vi "Auto_timed_strafe.vi"(3 "Strafe Speed":dbl, 4 "Strafe Time":dbl, 5 "RobotDriveDevRef in":T1) -> (2 "RobotDriveDevRef out":T1)   [LabVIEW 2017]
uses:
  <vilib>/Rock Robotics/WPI/RobotDrive/WPI_RobotDriveDevRef.ctl
  <vilib>/Rock Robotics/WPI/MotorControl/WPI_MotorControlDeviceRef.ctl
  <vilib>/Rock Robotics/WPI/MotorControl/WPI_MotorControlType.ctl
  <vilib>/Rock Robotics/SystemInterfaces/DIO/FPGA_DIOPWMChannel.ctl
  <vilib>/Rock Robotics/WPI/PWM/WPI_PWMDeadband.ctl
  <vilib>/Rock Robotics/SystemInterfaces/DIO/FPGA_DIOChannel.ctl
  <vilib>/Rock Robotics/WPI/RobotDrive/WPI_RobotDriveArcadeDrive_Standard(NoSaturation).vi
  <vilib>/Rock Robotics/Network Tables/NT Write Number.vi
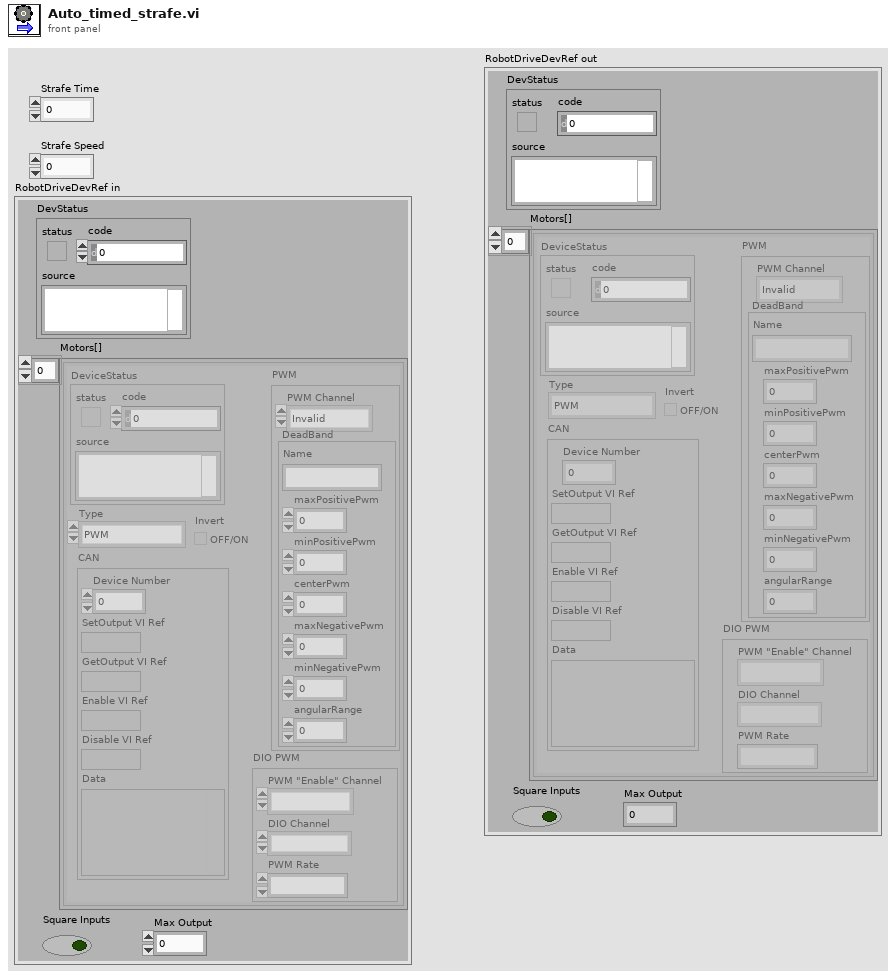
[diagram p1: front panel]
types:
  T1 = typedef "WPI_RobotDriveDevRef.ctl" = cluster{"DevStatus":errorcluster, "Motors[]":T2[], "Square Inputs":bool, "Max Output":dbl}
  T2 = typedef "WPI_MotorControlDeviceRef.ctl" = cluster{"DeviceStatus":errorcluster, "Type":T3, "PWM":cluster{"PWM Channel":T4, "DeadBand":T5}, "CAN":cluster{"Device Number":u8, "SetOutput VI Ref":variant, "GetOutput VI Ref":variant, "Enable VI Ref":variant, "Disable VI Ref":variant, "Data":variant}, "Invert":bool, "DIO PWM":cluster{"PWM \"Enable\" Channel":T4, "DIOChannel":T6, "PWM Rate":dbl}}
  T3 = typedef "WPI_MotorControlType.ctl" = enum16{"PWM", "CAN", "DIO PWM"}
  T4 = typedef "FPGA_DIOPWMChannel.ctl" = enum8{"PWM 0", "PWM 1", "PWM 2", "PWM 3", "PWM 4", "PWM 5", "PWM 6", "PWM 7", "PWM 8", "PWM 9", "PWM MXP 0", "PWM MXP 1", "PWM MXP 2", "PWM MXP 3", "PWM MXP 4", "PWM MXP 5", "PWM MXP 6", "PWM MXP 7", "PWM MXP 8", "PWM MXP 9", "Invalid"}
  T5 = typedef "WPI_PWMDeadband.ctl" = cluster{"Name":string, "maxPositivePwm":i32, "minPositivePwm":i32, "centerPwm":i32, "maxNegativePwm":i32, "minNegativePwm":i32, "angularRange":u16}
  T6 = typedef "FPGA_DIOChannel.ctl" = enum8{"DIO 0", "DIO 1", "DIO 2", "DIO 3", "DIO 4", "DIO 5", "DIO 6", "DIO 7", "DIO 8", "DIO 9", "DIO MXP 0", "DIO MXP 1", "DIO MXP 2", "DIO MXP 3", "DIO MXP 4", "DIO MXP 5", "DIO MXP 6", "DIO MXP 7", "DIO MXP 8", "DIO MXP 9", "DIO MXP 10", "DIO MXP 11", "DIO MXP 12", "DIO MXP 13", "DIO MXP 14", "DIO MXP 15", "SPI Port CS1", "SPI Port CS2", "SPI Port CS3", "SPI Port MISO", "SPI Port MOSI", "Invalid"}
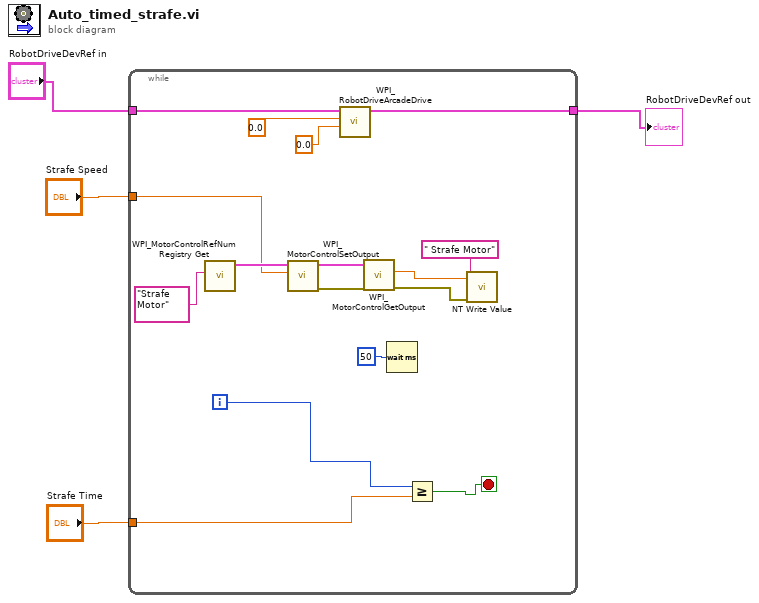
[diagram p0: block diagram]
diagram:
  n1 = while {
    tunnel: "Strafe Speed" -> [w11]
    tunnel: "Strafe Time" -> [w9]
    tunnel: "RobotDriveDevRef in" -> [w6]
    tunnel: [w5] -> w1
    i -> [w10]
    stop <- w20 stop-if-true
    n2 = call <vilib>:"WPI_MotorControlRefNum Registry Get.vi"("refnum name"="Strafe Motor") -> ("MotorControlDevRef"=w17:T2)  [unwired: 9 in, 1 out]
    n3 = call <vilib>:"WPI_MotorControlSetOutput.vi"("Output"=w11, "MotorControlDevRef"=w17) -> ("error out"=w15:errorcluster, "MotorControlDevRef"=w16:T2)  [unwired: 7 in, 1 out]
    n4 = call-poly <vilib>:"WPI_RobotDriveArcadeDrive.vi"("Y axis value"=0.0 ("X axis value"), "X axis value"=0.0, "RobotDriveDevRef"=w6) -> ("RobotDriveDevRef"=w5:T1)  [unwired: 1 in, 7 out]
    n5 = call <vilib>:"WPI_MotorControlGetOutput.vi"("error in (no error)"=w15, "MotorControlDevRef"=w16) -> ("error out"=w13:errorcluster, "Output"=w12:dbl)  [unwired: 7 in, 1 out]
    n6 = Wait (ms)(milliseconds to wait=50) -> ()  [unwired: 1 out]
    n7 = Greater Or Equal?(x=w10, y=w9) -> (x >= y?=w20:bool)
    n8 = call-poly <vilib>:"NT Write Value.vi"("error in"=w13, "Numeric"=w12, "Name"=" Strafe Motor") -> ()  [unwired: 8 in, 1 out]
  }
  "RobotDriveDevRef out" <- w1
